vi "RunByValue.vi"(8 "error in (no error)":errorcluster, 10 "BW icon in":T1, 11 "Color icon in":T1) -> (0 "error out":errorcluster, 1 "BW icon out":T1, 2 "Color icon out":T1, 3 "Error code out":i32)   [LabVIEW 2021, in "IconEditorInterface.lvlib" / "IconEditorInterface.lvclass"]
uses:
  <resource>/plugins/NIIconEditor/UI/Interface class/IconEditorInterface.lvclass
  <vilib>/picture/picture.llb/imagedata.ctl
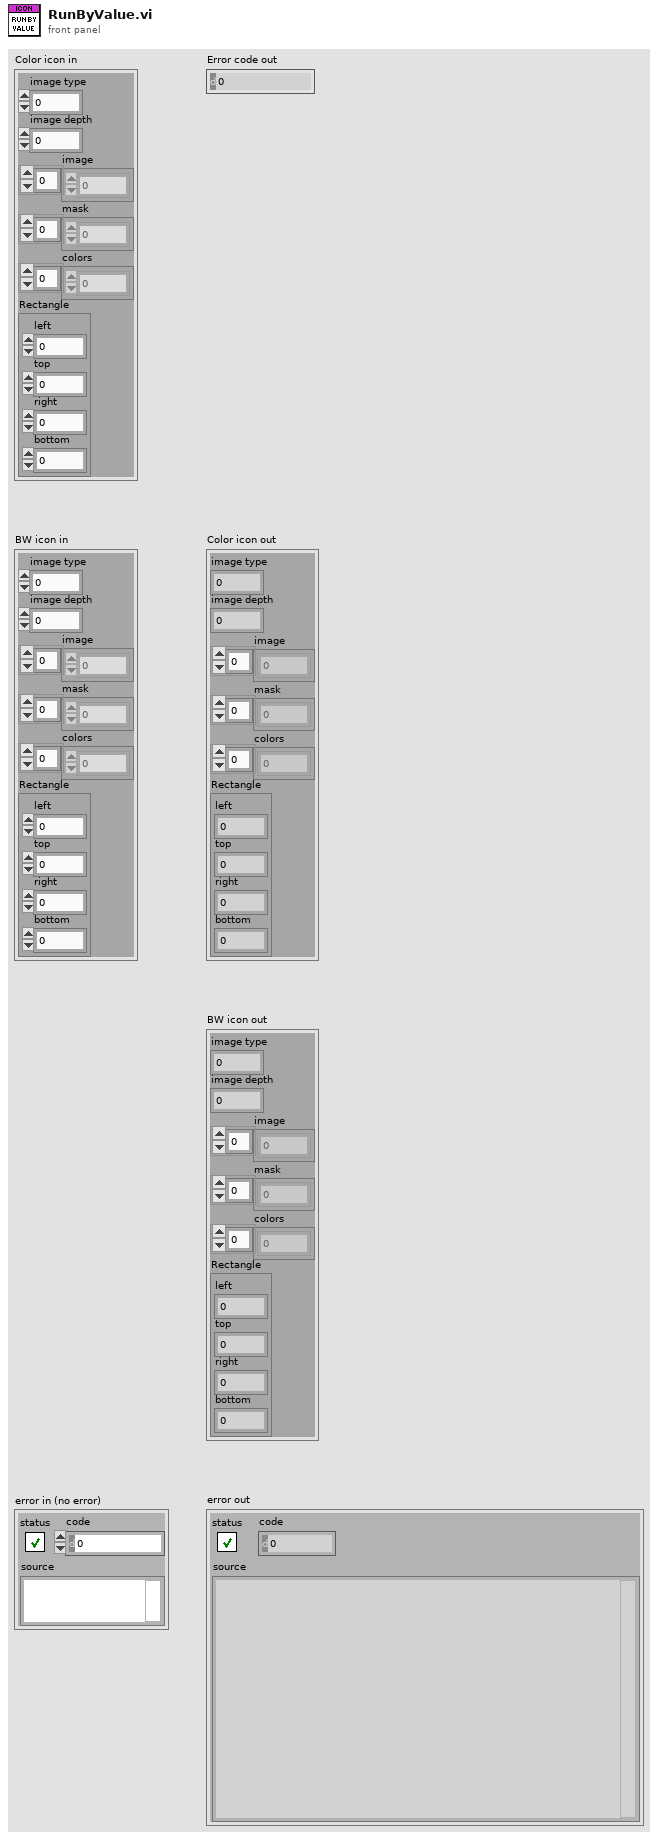
[diagram p1: front panel]
types:
  T1 = typedef "imagedata.ctl" = cluster{"image type":i32, "image depth":i32, "image":u8[], "mask":u8[], "colors":u32[], "Rectangle":cluster{"left":i16, "top":i16, "right":i16, "bottom":i16}}
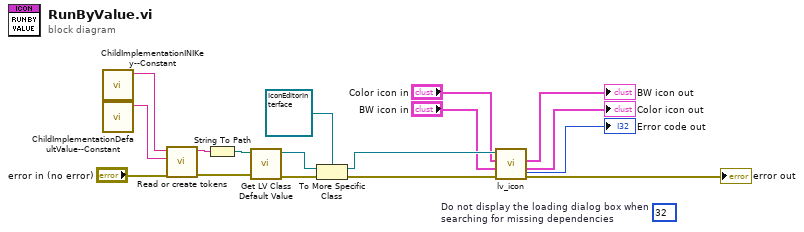
[diagram p0: block diagram]
diagram:
  (unwired) u32 32  # Do not display the loading dialog box when searching for missing dependencies
  n1 = call <resource>:"ChildImplementationINIKey--Constant.vi"() -> ("ChildImplementationPathKey"=w6:string)  [unwired: 11 in]
  n2 = call <resource>:"ChildImplementationDefaultValue--Constant.vi"() -> ("ChildImplementationDefaultValue"=w5:string)  [unwired: 11 in]
  n3 = call <resource>:"Read or create tokens.vi"("error in"="error in (no error)", "default value"=w5, "key"=w6) -> ("error out"=w3:errorcluster, "value"=w2:string)  [unwired: 7 in]
  n4 = String To Path(string=w2) -> (path=w1:path)
  n5 = call <vilib>:"Get LV Class Default Value.vi"("error in (no error)"=w3, "class path"=w1) -> ("error out"=w15:errorcluster, "object"=w17:refnum<class>)  [unwired: 8 in]
  n6 = To More Specific Class(target class=refnum<class "IconEditorInterface.lvclass"> refnum ("_IconEditorInterface.lvlib:_IconEditorInterface.lvclass"), reference=w17, error in=w15) -> (specific class reference=w12:refnum<class "IconEditorInterface.lvclass">, error out=w13:errorcluster)
  n7 = call-dynamic "lv_icon.vi"("error in (no error)"=w13, "BW icon in"="BW icon in", "Color icon in"="Color icon in", "_IconEditorInterface in"=w12) -> ("error out"=→"error out":errorcluster, "Color icon out"=→"Color icon out":T1, "BW icon out"=→"BW icon out":T1, "Error code out"=→"Error code out":i32)  [unwired: 3 in, 1 out]
